vi "call vi dynamically.vi"   [LabVIEW 2020, in "Reusable Library.lvlib"]
uses:
  Reusable Library.lvlib
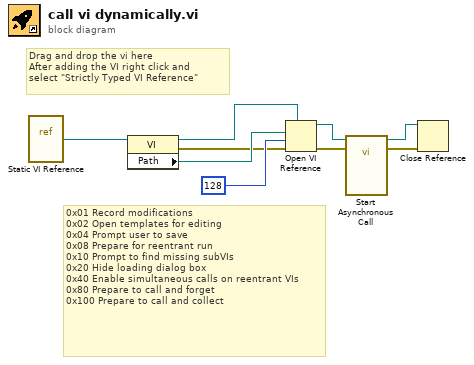
[diagram p0: block diagram]
diagram:
  # "0x01 Record modifications \n0x02 Open templates for editing\n0x04 Prompt user to save \n0x08 Prepare for reentrant run \n0x10 Prompt to find missing subVIs \n0x20 Hide loading dialog box\n0x40 Enable simultaneous calls on reentrant VIs  \n0x80 Prepare to call and forget \n0x100 Prepare to call and collect"
  # "Drag and drop the vi here\nAfter adding the VI right click and \nselect \"Strictly Typed VI Reference\""
  n1 = vi-ref "Static VI Reference"() -> ("vi reference"=w1:refnum<vi>)
  n2 = property class="VI"(reference=w1) -> (reference out=w8:refnum<vi>, error out=w4:errorcluster, "Path"=w9:path)  [unwired: 1 in]
  n3 = Open VI Reference(type specifier VI Refnum (for type only)=w8, vi path=w9, options=128, error in (no error)=w4) -> (vi reference=w2:refnum<vi>, error out=w5:errorcluster)  [unwired: 2 in]
  n4 = call-by-ref "Start Asynchronous Call"(reference=w2, error in=w5) -> (reference out=w3:refnum<vi>, error out=w6:errorcluster)  [unwired: 9 in, 3 out]
  n5 = Close Reference(reference=w3, error in (no error)=w6) -> ()  [unwired: 1 out]
